vi "Cluster.vi"() -> ()   [LabVIEW 2021]
panel:
  out "Modified Cluster":T1 {"Slide" scale=0.0..10.0}
  out "Small Cluster":cluster{"Slide Value":dbl, "Boolean1":bool}
  out "Boolean 2":bool
  in  "stop":bool
  out "Numeric":dbl
  in  "Cluster":T2 {"Slide" scale=0.0..10.0}
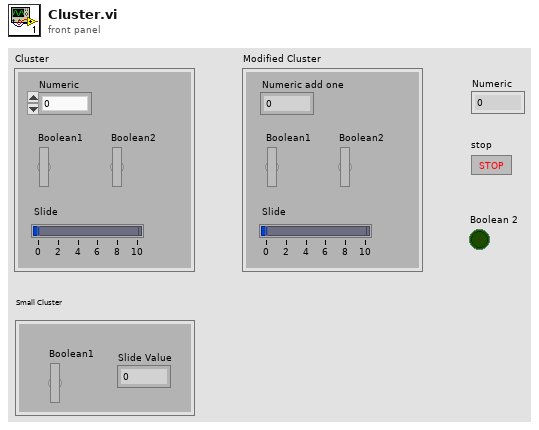
[diagram p1: front panel]
types:
  T1 = cluster{"Boolean1":bool, "Boolean2":bool, "Numeric add one":dbl, "Slide":dbl}
  T2 = cluster{"Boolean1":bool, "Boolean2":bool, "Numeric":dbl, "Slide":dbl}
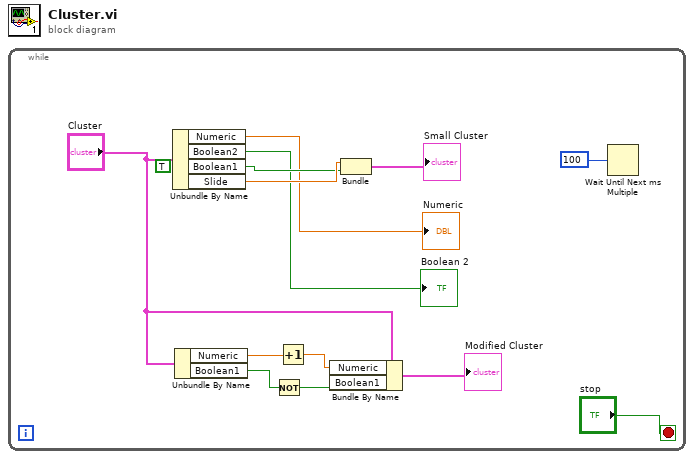
[diagram p0: block diagram]
diagram:
  n1 = while {
    stop <- "stop" stop-if-true
    (unwired) TRUE ("Boolean")
    n2 = Unbundle By Name("Cluster") -> ("Numeric"=→"Numeric":dbl, "Boolean2"=→"Boolean 2":bool, "Boolean1"=w9:bool, "Slide"=w10:dbl)
    n3 = Unbundle By Name("Cluster") -> ("Numeric"=w5:dbl, "Boolean1"=w7:bool)
    n4 = Not(x=w7) -> (.not. x?=w3:bool)
    n5 = Increment(x=w5) -> (x+1=w4:dbl)
    n6 = Bundle By Name(cluster="Cluster", "Numeric"=w4, "Boolean1"=w3) -> (→"Modified Cluster":T2)
    n7 = Bundle("Slide"=w10, "Boolean1"=w9) -> (→"Small Cluster":cluster{"Slide":dbl, "Boolean1":bool})  [unwired: 1 in]
    n8 = Wait Until Next ms Multiple(millisecond multiple=100) -> ()  [unwired: 1 out]
  }
